vi "Write Items.vi"(8 "error in (no error)":errorcluster, 10 "Items[]":string[](array[string]), 11 "OrderSelection in":refnum<class "OrderSelection.lvclass">) -> (0 "error out":errorcluster, 3 "OrderSelection out":refnum<class "OrderSelection.lvclass">)   [LabVIEW 2015, in "OrderSelection.lvclass"]
uses:
  OrderSelection.lvclass
  OrderSelection.lvclass/OrderSelection.ctl
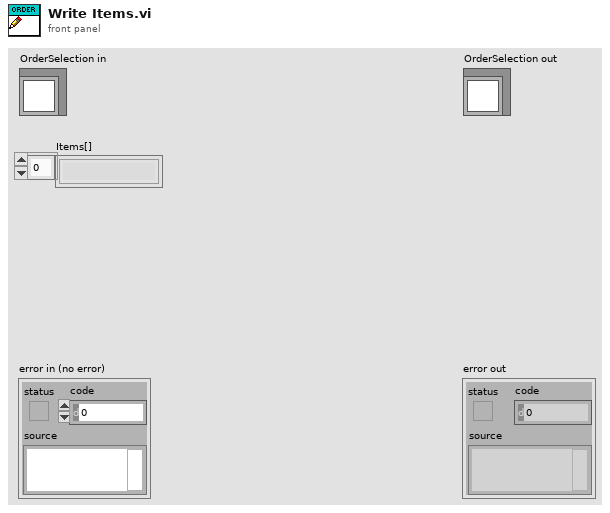
[diagram p1: front panel]
types:
  T1 = typedef "OrderSelection.lvclass/State Data.ctl" = cluster{"Items[]":string[], "SelectedItem":i32, "Position":i32, "ItemGraphic":T2}
  T2 = typedef "imagedata.ctl" = cluster{"image type":i32, "image depth":i32, "image":u8[], "mask":u8[], "colors":u32[], "Rectangle":cluster{"left":i16, "top":i16, "right":i16, "bottom":i16}}
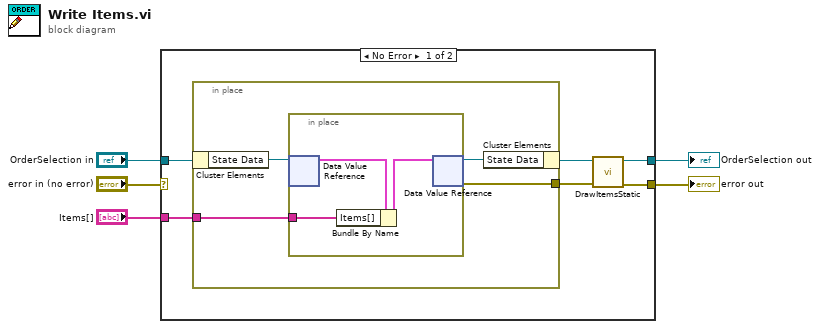
[diagram p0: block diagram]
diagram:
  n1 = case shown="No Error" "error in (no error)" {
    selector: "error in (no error)" -> [_ w20]
    tunnel: [w8 w20] -> w4
    tunnel: [w9 w19] -> w2
    tunnel: "OrderSelection in" -> [w11 w19]
    tunnel: "Items[]" -> [w10 _]
    frame No Error {
      n2 = in-place {
        in-place-border: w10 -> [w14]
        in-place-border: [w12] -> w6
        n3 = in-place-cluster #1(w11) -> ("State Data"=w15:refnum<data-value>)
        n4 = in-place {
          in-place-border: w14 -> [w17]
          n5 = in-place-dvr #2(w15) -> (w18:T1)  [unwired: 1 out]
          n6 = Bundle By Name(cluster=w18, "Items[]"=w17) -> (w16:T1)
          n7 = in-place-dvr #2(w16) -> (w13:refnum<data-value>, w12:errorcluster)
        }
        n8 = in-place-cluster #1("State Data"=w13) -> (w7:refnum<class "OrderSelection.lvclass">)
      }
      n9 = call "DrawItemsStatic.vi"("error in (no error)"=w6, "OrderSelection in"=w7) -> ("error out"=w8:errorcluster, "OrderSelection out"=w9:refnum<class "OrderSelection.lvclass">)  [unwired: 8 in]
    }
    frame Error {
    }
  }
  "error out" <- w4
  "OrderSelection out" <- w2
